vi "LNAttenuation.vi"(0 "index (row)":i32, 5 "data":dbl[][](array[numeric]), 9 "Upper Threshold (% of Max)":dbl=80.0, 11 "Lower Threshold (% of Min)":dbl=120.0) -> (4 "Upper Voltage Threshold Signal":dbl, 6 "Lower Voltage Threshold Signal":dbl, 8 "Upper Voltage Threshold Ref":dbl, 10 "LN Attenuation":dbl, 15 "Lower Voltage Threshold Ref":dbl)   [LabVIEW 2009]
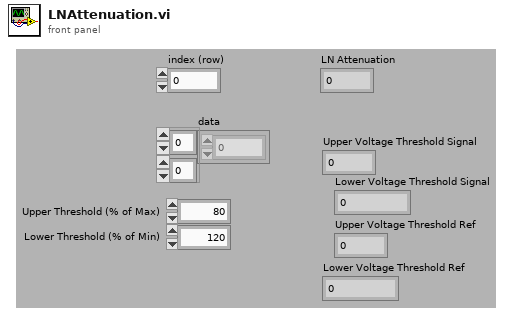
[diagram p1: front panel]
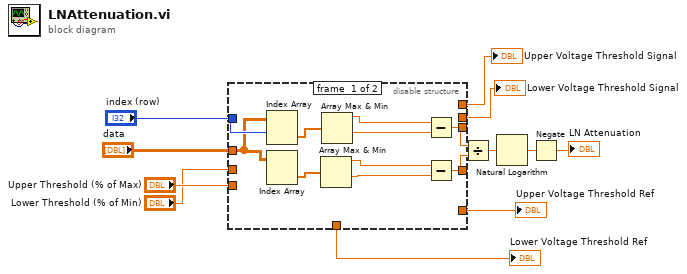
[diagram p0: block diagram]
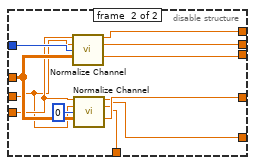
[diagram p2: hidden frame]
diagram:
  n1 = disable-structure shown="Enabled" {
    disable-tunnel: [w23 w31] -> w10
    disable-tunnel: [w22 w32] -> w9
    disable-tunnel: "index (row)" -> [w21 w34]
    disable-tunnel: "data" -> [w14 w33]
    disable-tunnel: "Upper Threshold (% of Max)" -> [_ w29]
    disable-tunnel: "Lower Threshold (% of Min)" -> [_ w28]
    disable-tunnel: [_ w27] -> w4
    disable-tunnel: [_ w26] -> w3
    disable-tunnel: [_ w25] -> w2
    disable-tunnel: [_ w24] -> w1
    frame #0 {
      n2 = Index Array(array=w14, index (row)=w21) -> (element=w16:dbl[])  [unwired: 1 in]
      n3 = Index Array(array=w14) -> (element=w15:dbl[])  [unwired: 2 in]
      n4 = Array Max & Min(array=w15) -> (max value=w20:dbl, min value=w19:dbl)  [unwired: 2 out]
      n5 = Array Max & Min(array=w16) -> (max value=w18:dbl, min value=w17:dbl)  [unwired: 2 out]
      n6 = Subtract(x=w18, y=w17) -> (x-y=w23:dbl)
      n7 = Subtract(x=w20, y=w19) -> (x-y=w22:dbl)
    }
    frame #1 {
      n8 = call "Normalize Channel.vi"("Upper Threshold (% of Max)"=w29, "Lower Threshold (% of Min)"=w28, "index (row)"=w34, "data"=w33) -> ("Upper Voltage Threshold"=w27:dbl, "Lower Voltage Threshold"=w25:dbl, "Normalized Max (Channel Max - Channel Min)"=w31:dbl)  [unwired: 7 in, 2 out]
      n9 = call "Normalize Channel.vi"("Upper Threshold (% of Max)"=w29, "Lower Threshold (% of Min)"=w28, "index (row)"=0, "data"=w33) -> ("Upper Voltage Threshold"=w26:dbl, "Lower Voltage Threshold"=w24:dbl, "Normalized Max (Channel Max - Channel Min)"=w32:dbl)  [unwired: 7 in, 2 out]
    }
  }
  "Upper Voltage Threshold Signal" <- w4
  "Lower Voltage Threshold Signal" <- w2
  "Upper Voltage Threshold Ref" <- w3
  "Lower Voltage Threshold Ref" <- w1
  n10 = Divide(x=w10, y=w9) -> (x/y=w11:dbl)
  n11 = Natural Logarithm(1:w11) -> (0:w12:dbl)
  n12 = Negate(x=w12) -> (-x=→"LN Attenuation":dbl)
